vi "new_CTR_DAQSensorConfigs.vi"(8 "error in":errorcluster, 10 "Sensors in":T1(array[cluster]), 11 "node in":refnum<k20>) -> (0 "error out":errorcluster={"status"=TRUE, "code"=-2633, "source"="Property Node (arg 1) in NI_XML.lvlib:Get Node Text Content.vi->CTR_ControlNodeConfigs.vi->CTR_ReadXML_Config.vi->CTRnode.vi"}, 2 "Sensors out":T1(array[cluster]), 3 "node out":refnum<k20>)   [LabVIEW 2024]
uses:
  <vilib>/xml/Close Reference(Node).vi
  <vilib>/xml/NI_XML.lvlib
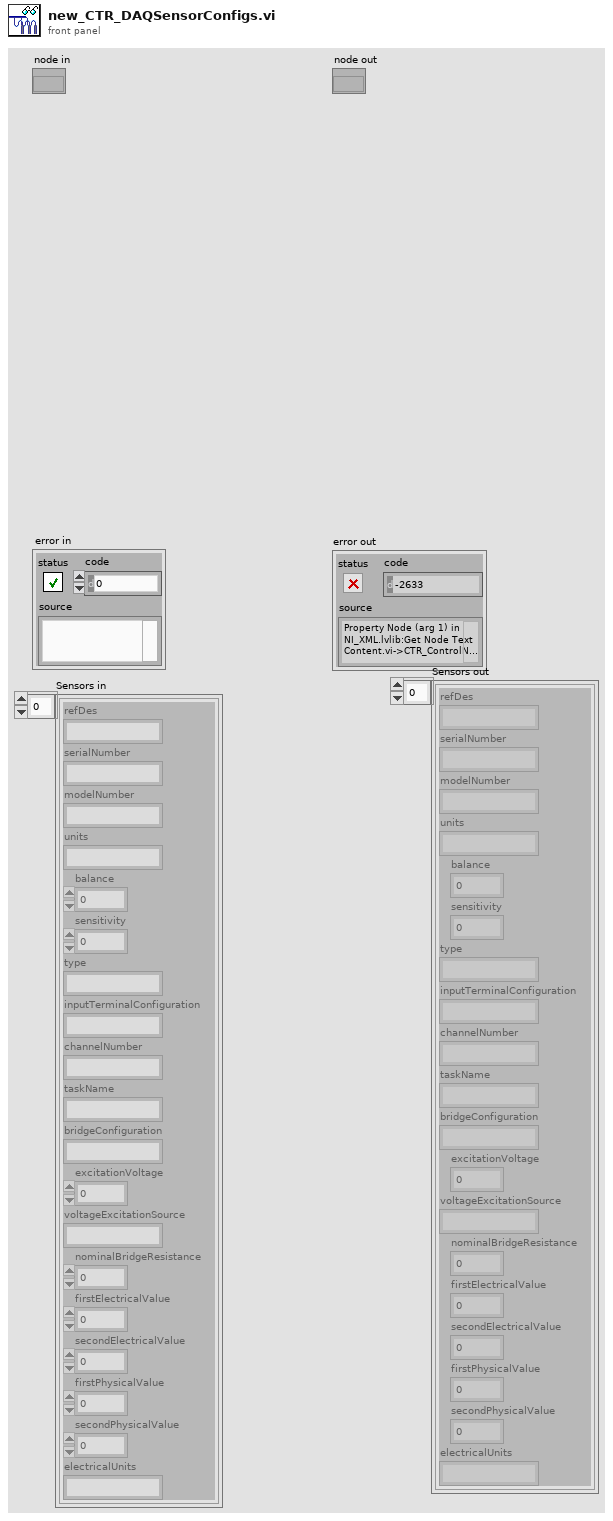
[diagram p1: front panel]
types:
  T1 = cluster{"refDes":string, "serialNumber":string, "modelNumber":string, "units":string, "balance":dbl, "sensitivity":dbl, "type":string, "inputTerminalConfiguration":string, "channelNumber":string, "taskName":string, "bridgeConfiguration":string, "excitationVoltage":dbl, "voltageExcitationSource":string, "nominalBridgeResistance":dbl, "firstElectricalValue":dbl, "secondElectricalValue":dbl, "firstPhysicalValue":dbl, "secondPhysicalValue":dbl, "electricalUnits":string}[]
  T2 = cluster{"refDes":string, "serialNumber":string, "modelNumber":string, "units":string, "balance":dbl, "sensitivity":dbl, "type":string, "inputTerminalConfiguration":string, "channelNumber":string, "taskName":string, "bridgeConfiguration":string, "excitationVoltage":dbl, "voltageExcitationSource":string, "nominalBridgeResistance":dbl, "firstElectricalValue":dbl, "secondElectricalValue":dbl, "firstPhysicalValue":dbl, "secondPhysicalValue":dbl, "electricalUnits":string}
  T3 = cluster{"[0]":string, "[1]":string, "[2]":string, "[3]":string, "[4]":string, "[5]":string, "[6]":string, "[7]":string, "[8]":string, "[9]":string, "[10]":string, "[11]":string, "[12]":string, "[13]":string, "[14]":string, "[15]":string, "[16]":string, "[17]":string, "[18]":string}
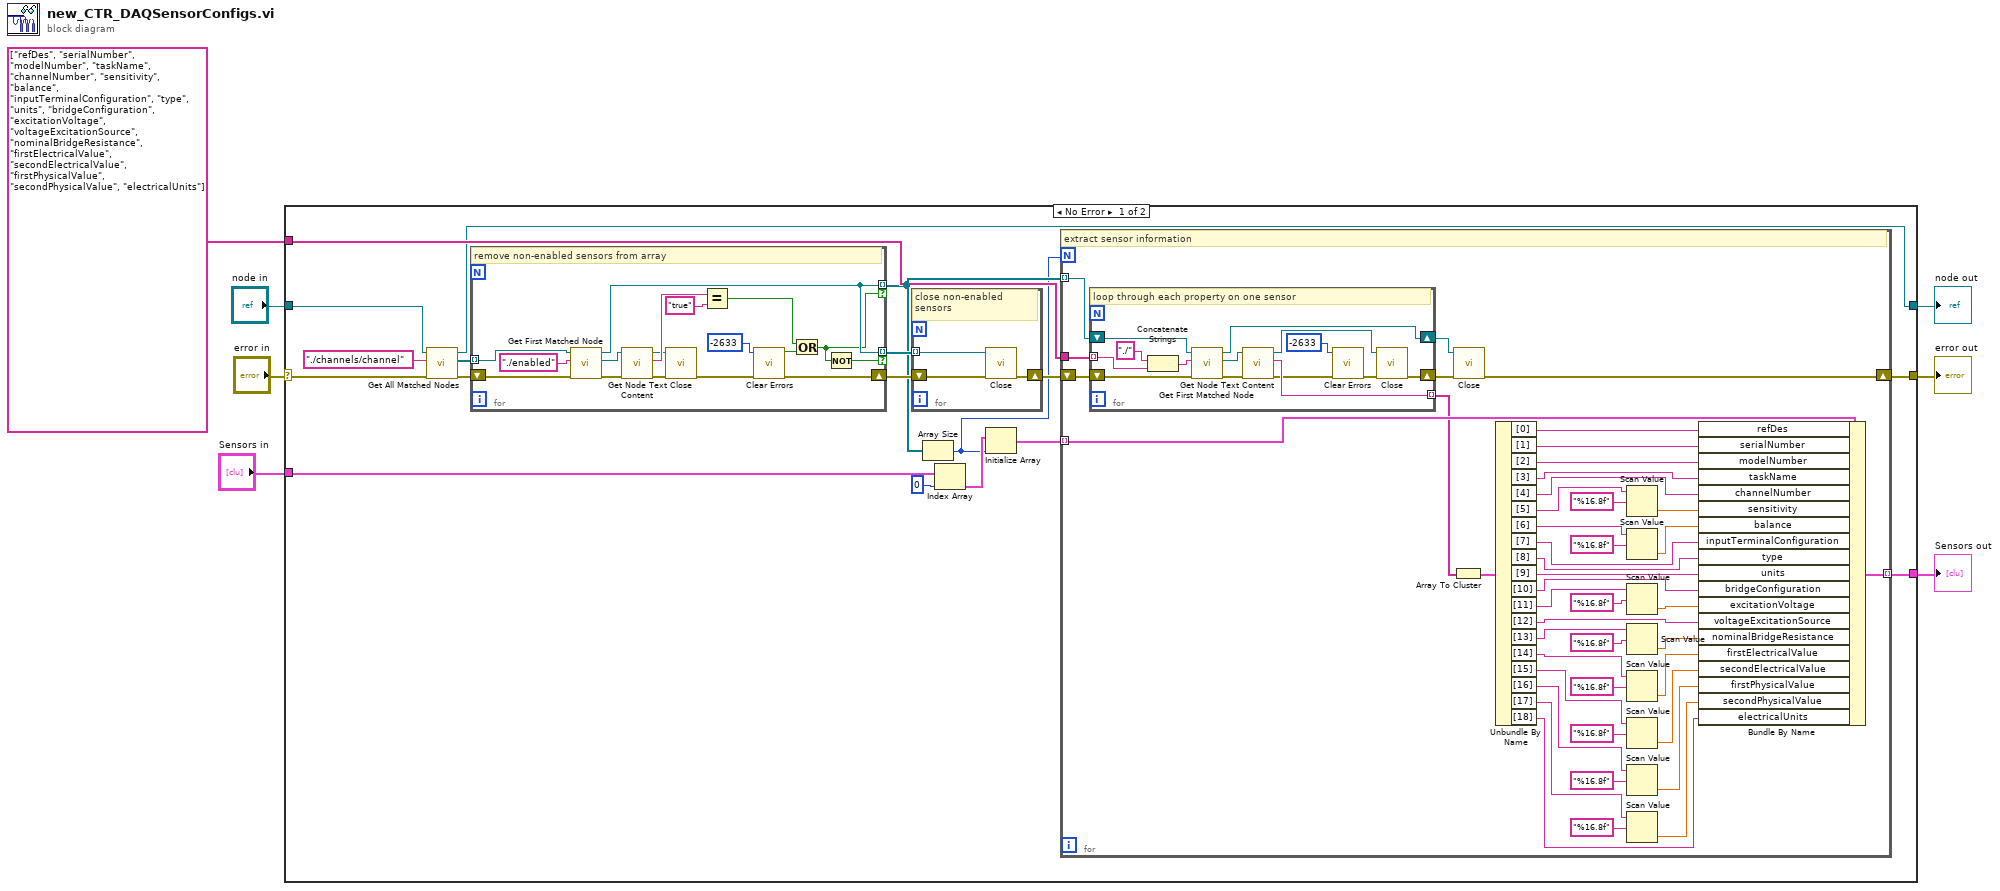
[diagram p0: block diagram]
diagram:
  n1 = case shown="No Error" "error in" {
    selector: "error in" -> [w25 w107]
    tunnel: [w24 w107] -> w6
    tunnel: "node in" -> [w22 w106]
    tunnel: string[] ["refDes", "serialNumber", "modelNumber", "taskName", "channelNumber", "sensitivity", "balance", "inputTerminalConfiguration", "type", "units", "bridgeConfiguration", "excitationVoltage", "voltageExcitationSource", "nominalBridgeResistance", "firstElectricalValue", "secondElectricalValue", "firstPhysicalValue", "secondPhysicalValue", "electricalUnits"] -> [w21 _]
    tunnel: [w13 w106] -> w7
    tunnel: "Sensors in" -> [w9 w105]
    tunnel: [w8 w105] -> w2
    frame No Error {
      n2 = call <vilib>:"Get All Matched Nodes.vi"("error in (no error)"=w25, "XPath expression"="./channels/channel" ("string"), "node in"=w22) -> ("error out"=w17:errorcluster, "node result array"=w14:refnum<k20>[], "node out"=w13:refnum<k20>)  [unwired: 6 in]
      n3 = for {
        shift-right: [w32] -> w19
        shift-left: w17 -> [w38]
        tunnel: [w37] -> w15 mode=indexing if=w29
        tunnel: [w37] -> w18 mode=indexing if=w36
        tunnel: w14 -> [w35] mode=indexing
        # "remove non-enabled sensors from array"
        n4 = call <vilib>:"Get First Matched Node.vi"("error in (no error)"=w38, "XPath expression"="./enabled", "node in"=w35) -> ("error out"=w41:errorcluster, "node result"=w42:refnum<k20>, "node out"=w37:refnum<k20>)  [unwired: 6 in]
        n5 = call <vilib>:"Get Node Text Content.vi"("error in (no error)"=w41, "node in"=w42) -> ("error out"=w43:errorcluster, "node text"=w45:string, "node out"=w44:refnum<k20>)  [unwired: 7 in]
        n6 = call-poly <vilib>:"Close.vi"("error in (no error)"=w43, "node"=w44) -> ("error out"=w33:errorcluster)  [unwired: 7 in]
        n7 = Equal?(x=w45, y="true" ("x")) -> (x = y?=w31:bool)
        n8 = call <vilib>:"Clear Errors.vi"("error in (no error)"=w33, "specific error code to clear (0: all)"=-2633) -> ("error out"=w32:errorcluster, "specific error cleared?"=w30:bool)  [unwired: 4 in]
        n9 = Or(x=w31, y=w30) -> (x .or. y?=w29:bool)
        n10 = Not(x=w29) -> (.not. x?=w36:bool)
      }
      n11 = for {
        tunnel: w18 -> [w28] mode=indexing
        shift-right: [w26] -> w16
        shift-left: w19 -> [w27]
        # "close non-enabled sensors"
        n12 = call-poly <vilib>:"Close.vi"("error in (no error)"=w27, "node"=w28) -> ("error out"=w26:errorcluster)  [unwired: 7 in]
      }
      n13 = Array Size(array=w15) -> (size(s)=w11:i32)
      n14 = Index Array(array=w9, index=0) -> (element=w12:T2)
      n15 = Initialize Array(w12, w11) -> (w10:T1)
      n16 = for {
        N: w11 -> [_]
        shift-right: [w73] -> w24
        shift-left: w16 -> [w89]
        tunnel: w21 -> [w90]
        tunnel: w15 -> [w88] mode=indexing
        tunnel: w10 -> [w87] mode=indexing
        tunnel: [w82] -> w8 mode=indexing
        # "extract sensor information"
        n17 = for {
          tunnel: w90 -> [w99] mode=indexing
          shift-right: [w94] -> w83
          shift-left: w89 -> [w101]
          shift-right: [w96] -> w84
          shift-left: w88 -> [w97]
          tunnel: [w95] -> w86 mode=indexing
          # "loop through each property on one sensor"
          n18 = Concatenate Strings("./" ("string"), w99) -> (w98:string)
          n19 = call <vilib>:"Get First Matched Node.vi"("error in (no error)"=w101, "XPath expression"=w98, "node in"=w97) -> ("error out"=w104:errorcluster, "node result"=w103:refnum<k20>, "node out"=w96:refnum<k20>)  [unwired: 6 in]
          n20 = call <vilib>:"Get Node Text Content.vi"("error in (no error)"=w104, "node in"=w103) -> ("error out"=w93:errorcluster, "node text"=w95:string, "node out"=w102:refnum<k20>)  [unwired: 7 in]
          n21 = call <vilib>:"Clear Errors.vi"("error in (no error)"=w93, "specific error code to clear (0: all)"=-2633) -> ("error out"=w92:errorcluster)  [unwired: 4 in, 1 out]
          n22 = call-poly <vilib>:"Close.vi"("error in (no error)"=w92, "node"=w102) -> ("error out"=w94:errorcluster)  [unwired: 7 out]
        }
        n23 = Array To Cluster(array=w86) -> (cluster=w85:T3)
        n24 = call-poly <vilib>:"Close.vi"("error in (no error)"=w83, "node"=w84) -> ("error out"=w73:errorcluster)  [unwired: 7 out]
        n25 = Unbundle By Name(w85) -> ("[0]"=w74:string, "[1]"=w75:string, "[2]"=w76:string, "[3]"=w77:string, "[4]"=w78:string, "[5]"=w72:string, "[6]"=w69:string, "[7]"=w79:string, "[8]"=w80:string, "[9]"=w81:string, "[10]"=w62:string, "[11]"=w53:string, "[12]"=w52:string, "[13]"=w51:string, "[14]"=w50:string, "[15]"=w49:string, "[16]"=w48:string, "[17]"=w47:string, "[18]"=w46:string)
        n26 = Scan Value(string=w72, format string="%16.8f") -> (value=w67:dbl)  [unwired: 1 in, 1 out]
        n27 = Scan Value(string=w69, format string="%16.8f") -> (value=w68:dbl)  [unwired: 1 in, 1 out]
        n28 = Scan Value(string=w53, format string="%16.8f") -> (value=w63:dbl)  [unwired: 1 in, 1 out]
        n29 = Scan Value(string=w51, format string="%16.8f") -> (value=w60:dbl)  [unwired: 1 in, 1 out]
        n30 = Scan Value(string=w50, format string="%16.8f") -> (value=w58:dbl)  [unwired: 1 in, 1 out]
        n31 = Scan Value(string=w49, format string="%16.8f") -> (value=w56:dbl)  [unwired: 1 in, 1 out]
        n32 = Scan Value(string=w48, format string="%16.8f") -> (value=w54:dbl)  [unwired: 1 in, 1 out]
        n33 = Scan Value(string=w47, format string="%16.8f") -> (value=w65:dbl)  [unwired: 1 in, 1 out]
        n34 = Bundle By Name(cluster=w87, "refDes"=w74, "serialNumber"=w75, "modelNumber"=w76, "taskName"=w77, "channelNumber"=w78, "sensitivity"=w67, "balance"=w68, "inputTerminalConfiguration"=w79, "type"=w80, "units"=w81, "bridgeConfiguration"=w62, "excitationVoltage"=w63, "voltageExcitationSource"=w52, "nominalBridgeResistance"=w60, "firstElectricalValue"=w58, "secondElectricalValue"=w56, "firstPhysicalValue"=w54, "secondPhysicalValue"=w65, "electricalUnits"=w46) -> (w82:T2)
      }
    }
    frame Error {
    }
  }
  "error out" <- w6
  "node out" <- w7
  "Sensors out" <- w2
